vi "HEWH Remove 5 Minutes.vi"(0 "Watt Hours":dbl[](array[numeric]), 1 "Elapsed Time (sec)":dbl[](array[numeric]), 5 "Energy (BTU)":dbl[](array[numeric]), 7 "TC Tree Average":dbl[](array[numeric]), 9 "Take5MinSample":u8, 11 "error in (no error)":errorcluster, 13 "Qr (T), SU0 (F)":bool=TRUE) -> (3 "Elapsed Time (sec) Sub Array":dbl[](array[numeric]), 4 "TC Tree Average Sub Array":dbl[](array[numeric]), 6 "Energy (BTU) Sub Array":dbl[](array[numeric]), 8 "5 Minute Subset Index Adder":i32, 10 "Watt Hour Sub Array":dbl[](array[numeric]), 15 "error out":errorcluster)   [LabVIEW 2023]
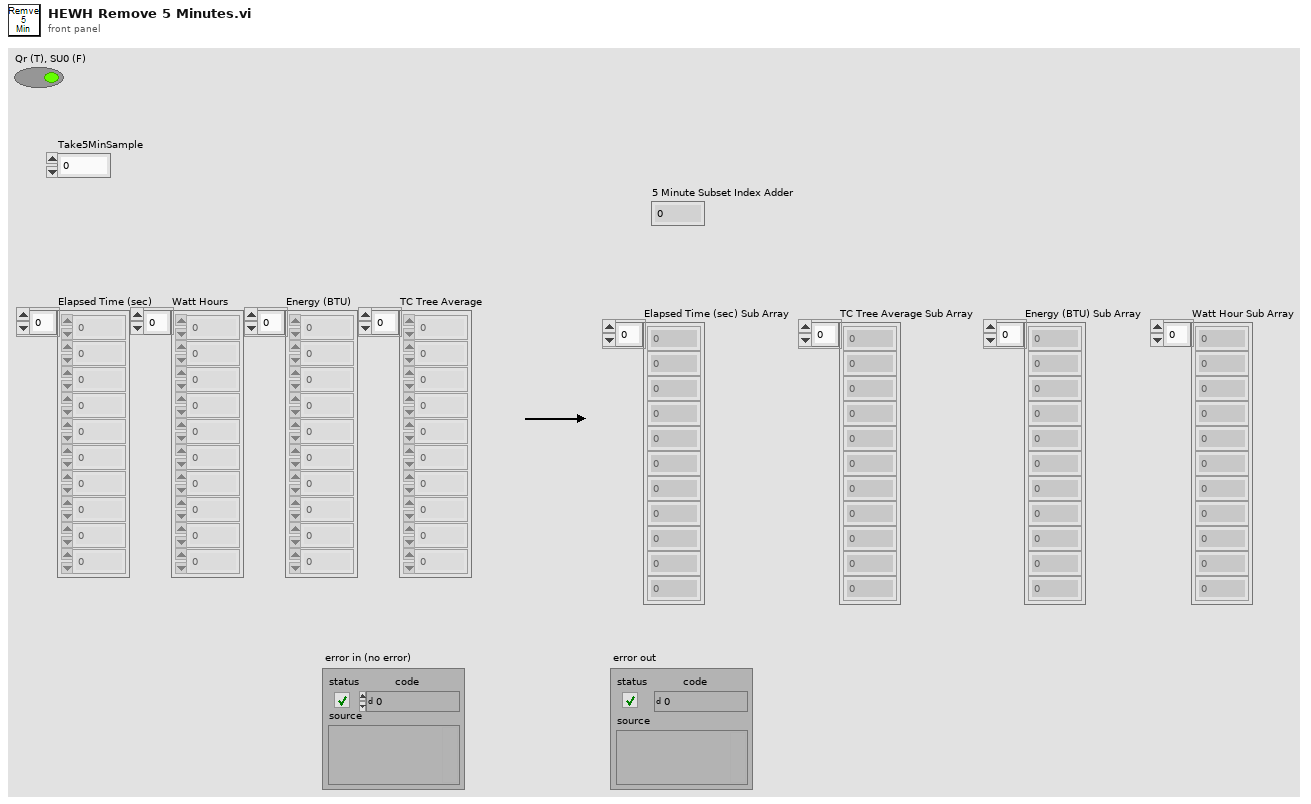
[diagram p1: front panel]
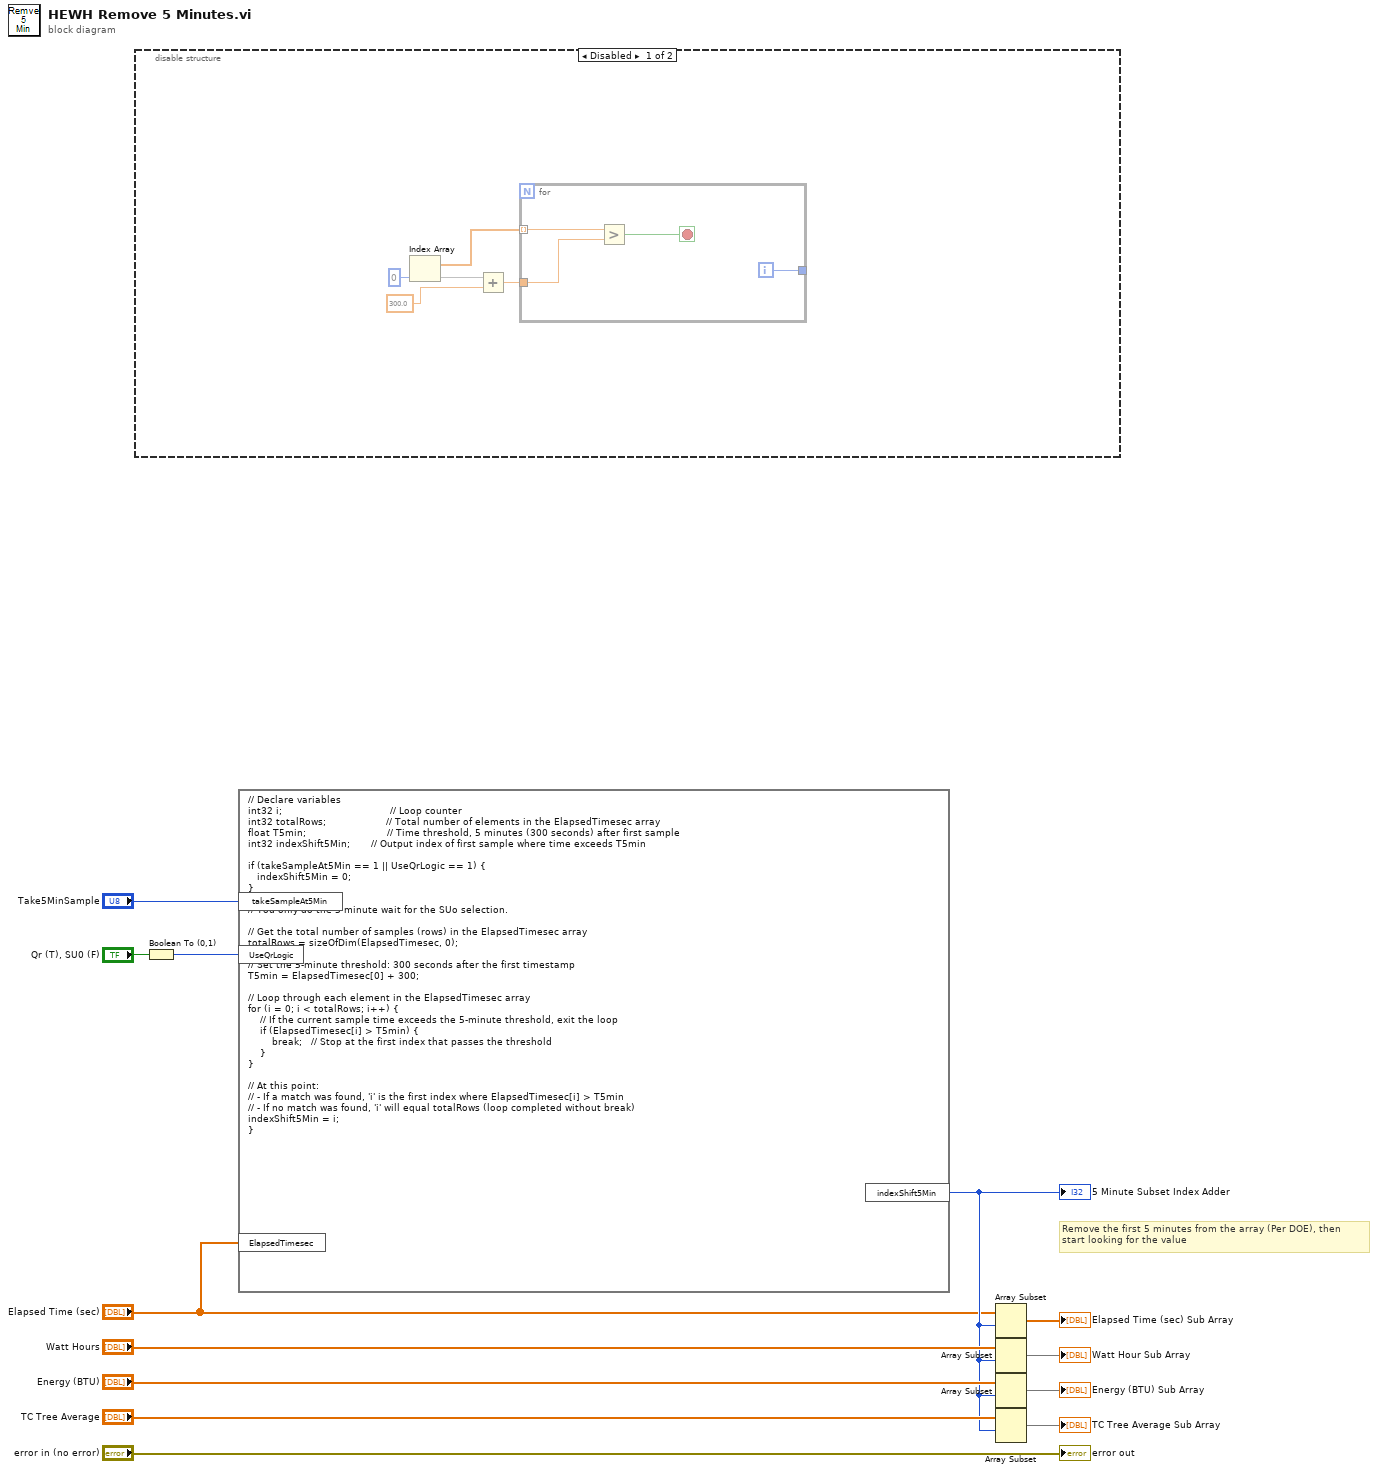
[diagram p0: block diagram]
diagram:
  # "Remove the first 5 minutes from the array (Per DOE), then \nstart looking for the value"
  n1 = disable-structure shown="Disabled" {
    frame Disabled {
      n2 = Index Array "Index Array"(array=w18, index=0) -> (element=w16)
      n3 = Add(x=w16, y=300.0) -> (x+y=w17:dbl)
      n4 = for {
        tunnel: [w22] -> w18 mode=indexing
        tunnel: w17 -> [w21]
        tunnel: [w19] -> _
        i -> [w19]
        stop <- w20 stop-if-true
        n5 = Greater?(x=w22, y=w21) -> (0:w20:bool)
      }
    }
    frame Enabled {
    }
  }
  n6 = Boolean To (0,1)(Boolean="Qr (T), SU0 (F)") -> (0, 1=w2:i16)
  n7 = formula code="// Declare variables\nint32 i;                                    // Loop counter\nint32 totalRows;                    // Total number of elements in the ElapsedTimesec array\nfloat T5min;                           // Time threshold, 5 minutes (300 seconds) after first sample\nint32 indexShift5Min;       // Output index of first sample where time exceeds T5min\n\nif (takeSampleAt5Min == 1 || UseQrLogic == 1) {\n   indexShift5Min = 0;\n}\nelse {\n// You only do the 5 minute wait for the SUo selection.\n\n// Get the total number of samples (rows) in the ElapsedTimesec array\ntotalRows = sizeOfDim(ElapsedTimesec, 0);\n\n// Set the 5-minute threshold: 300 seconds after the first timestamp\nT5min = ElapsedTimesec[0] + 300;\n\n// Loop through each element in the ElapsedTimesec array\nfor (i = 0; i < totalRows; i++) {\n    // If the current sample time exceeds the 5-minute threshold, exit the loop\n    if (ElapsedTimesec[i] > T5min) {\n        break;   // Stop at the first index that passes the threshold\n    }\n}\n\n// At this point:\n// - If a match was found, 'i' is the first index where ElapsedTimesec[i] > T5min\n// - If no match was found, 'i' will equal totalRows (loop completed without break)\nindexShift5Min = i;\n}"("ElapsedTimesec"="Elapsed Time (sec)", "takeSampleAt5Min"="Take5MinSample", "UseQrLogic"=w2) -> ("indexShift5Min"=w5:i32)
  "5 Minute Subset Index Adder" <- w5
  n8 = Array Subset(array="Elapsed Time (sec)", index=w5) -> (→"Elapsed Time (sec) Sub Array":dbl[])  [unwired: 1 in]
  n9 = Array Subset(array="Watt Hours", index=w5) -> (→"Watt Hour Sub Array":dbl[])  [unwired: 1 in]
  n10 = Array Subset(array="Energy (BTU)", index=w5) -> (→"Energy (BTU) Sub Array":dbl[])  [unwired: 1 in]
  n11 = Array Subset(array="TC Tree Average", index=w5) -> (→"TC Tree Average Sub Array":dbl[])  [unwired: 1 in]
  "error out" <- "error in (no error)"
